vi "Initialize.vi"(8 "error in (no error)":errorcluster, 11 "State in":T1={"State"=enum."Idle", "Start Time"=timestamp(0 s since 1904-01-01), "Configuration"={"Cycle Period"=0.0, "PID 2 Parameters"={"Input Device"=enum."4-20mA", "Output Device"=enum."Default", "Setpoint"=0.0, "PID gains"={"proportional gain (Kc)"=0.0, "integral time (Ti, min)"=0.0, "derivative time (Td, min)"=100.0}, "output range"={"output low"=0.0, "output high"=1.0}}, "Manual Entry"=0.0, "Auto?"=TRUE, "4-20mA Input Settings"={"Input Channel "=0}, "4-20mA Out Settings"={"Output DAQ Task"=""}, "Input Channel Tag Name "=""}, "Current Time"=timestamp(0 s since 1904-01-01), "PID 1 Parameters"={"Setpoint"=0.0, "PID gains"={"proportional gain (Kc)"=1.0, "integral time (Ti, min)"=0.01, "derivative time (Td, min)"=0.0}}, "First Iteration"=FALSE, "Data"={"4-20mA Input"=0.0, "PID 2 Process Variable"=0.0, "PID 2 Output"=0.0, "4-20mA Output"=0.0}, "Process Name"="", "Pump On?"=enum."Off", "Input Error"=FALSE, "Output Error"=FALSE, "Log Started"=FALSE, "Current Setpoint"=0.0} {"Configuration"."PID 2 Parameters"."output range"."output low" format="%.2f"; "Configuration"."PID 2 Parameters"."output range"."output high" min=0.0 max=100.0 format="%.2f"; "Configuration"."PID 2 Parameters"."PID gains"."derivative time (Td, min)" format="%.3f"; "Configuration"."PID 2 Parameters"."PID gains"."integral time (Ti, min)" format="%.3f"; "Configuration"."PID 2 Parameters"."PID gains"."proportional gain (Kc)" format="%.3f"; "PID 1 Parameters"."PID gains"."derivative time (Td, min)" format="%.3f"; "PID 1 Parameters"."PID gains"."integral time (Ti, min)" format="%.3f"; "PID 1 Parameters"."PID gains"."proportional gain (Kc)" format="%.3f"}) -> (0 "error out":errorcluster, 1 "Pump Initialized":bool, 3 "State out":T1={"State"=enum."Idle", "Start Time"=timestamp(0 s since 1904-01-01), "Configuration"={"Cycle Period"=0.0, "PID 2 Parameters"={"Input Device"=enum."4-20mA", "Output Device"=enum."Default", "Setpoint"=0.0, "PID gains"={"proportional gain (Kc)"=0.0, "integral time (Ti, min)"=0.0, "derivative time (Td, min)"=100.0}, "output range"={"output low"=0.0, "output high"=1.0}}, "Manual Entry"=0.0, "Auto?"=TRUE, "4-20mA Input Settings"={"Input Channel "=0}, "4-20mA Out Settings"={"Output DAQ Task"=""}, "Input Channel Tag Name "=""}, "Current Time"=timestamp(0 s since 1904-01-01), "PID 1 Parameters"={"Setpoint"=0.0, "PID gains"={"proportional gain (Kc)"=1.0, "integral time (Ti, min)"=0.01, "derivative time (Td, min)"=0.0}}, "First Iteration"=FALSE, "Data"={"4-20mA Input"=0.0, "PID 2 Process Variable"=0.0, "PID 2 Output"=0.0, "4-20mA Output"=0.0}, "Process Name"="", "Pump On?"=enum."Off", "Input Error"=FALSE, "Output Error"=FALSE, "Log Started"=FALSE, "Current Setpoint"=0.0} {"Configuration"."PID 2 Parameters"."output range"."output low" format="%.2f"; "Configuration"."PID 2 Parameters"."output range"."output high" min=0.0 max=100.0 format="%.2f"; "Configuration"."PID 2 Parameters"."PID gains"."derivative time (Td, min)" format="%.3f"; "Configuration"."PID 2 Parameters"."PID gains"."integral time (Ti, min)" format="%.3f"; "Configuration"."PID 2 Parameters"."PID gains"."proportional gain (Kc)" format="%.3f"; "PID 1 Parameters"."PID gains"."derivative time (Td, min)" format="%.3f"; "PID 1 Parameters"."PID gains"."integral time (Ti, min)" format="%.3f"; "PID 1 Parameters"."PID gains"."proportional gain (Kc)" format="%.3f"})   [LabVIEW 2018, in "4-20mA Module.lvlib" / "4-20mA Module Engine.lvlib"]
uses:
  4-20mA Module Engine.lvlib
  State Cluster.ctl
  State Enum.ctl
  Pressure Transmitter/Pressure Transmitter Device Settings.ctl
  Pressure Reg Module/Pressure Regulator Device Settings.ctl
  Measure Instrument/PID 1 Parameters Cluster.ctl
  Tag VIs/Tag FGV Operation Enum.ctl
  Shared Variables/Dynamic Shared Variables.lvlib
  Pressure Transmitter/Pressure Transmitter Library.lvlib
  Pressure Reg Module/Pressure Regulator Library.lvlib
panel:
  # "Instrument Settings"
  # "Instrument Settings"
  # "Instrument Settings"
  # "Instrument Settings"
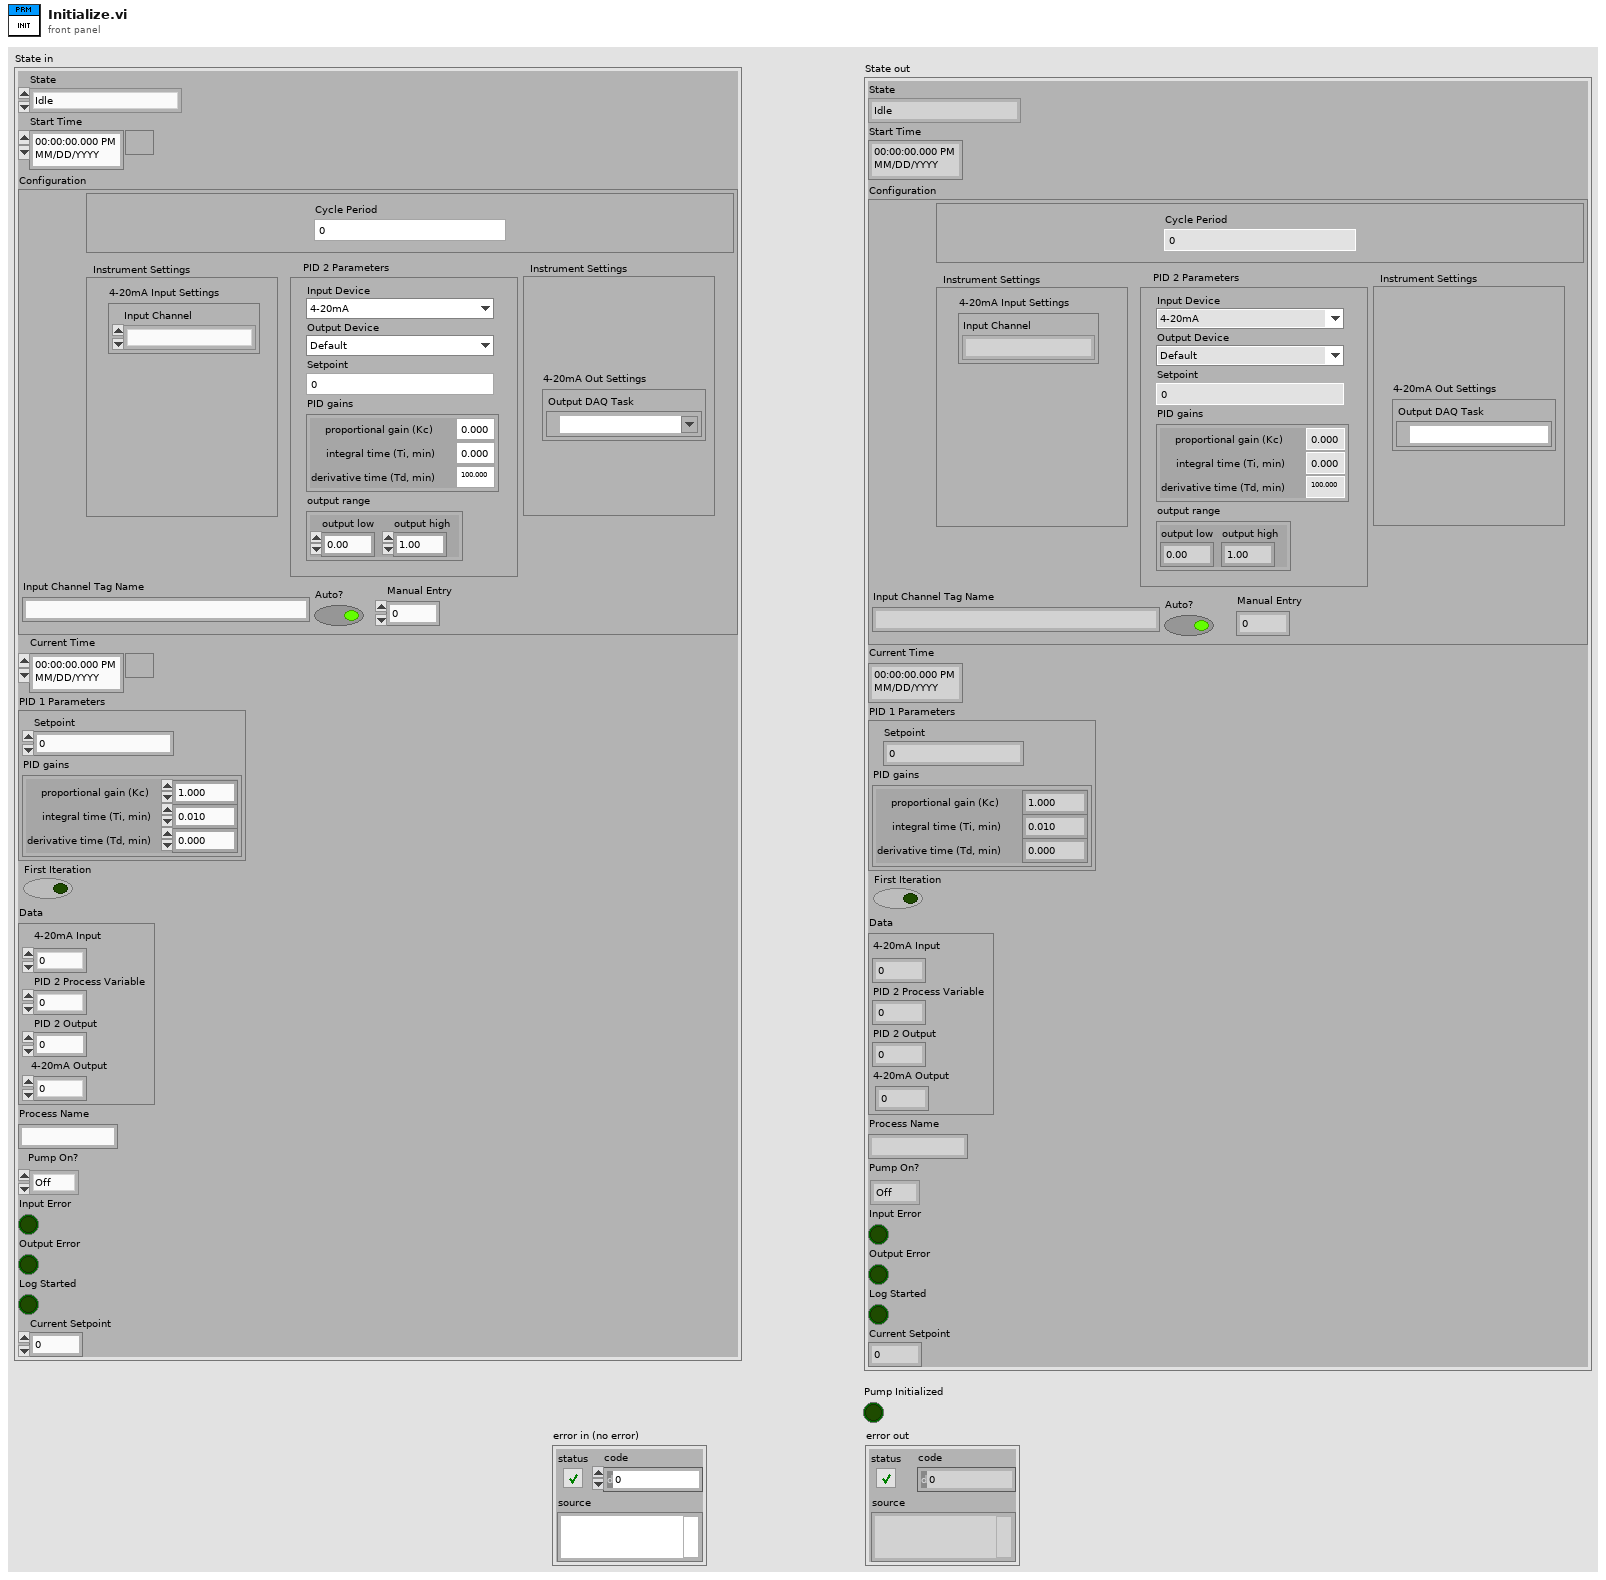
[diagram p1: front panel]
types:
  T1 = typedef "4-20mA Module.lvlib/4-20mA Module Engine.lvlib/State Cluster.ctl" = cluster{"State":T2, "Start Time":timestamp, "Configuration":cluster{"Cycle Period":dbl, "PID 2 Parameters":cluster{"Input Device":enum16{"Default", "4-20mA"}, "Output Device":enum16{"Default", "Equilibar Pressure Reg", "Flow Regulator"}, "Setpoint":dbl, "PID gains":cluster{"proportional gain (Kc)":dbl, "integral time (Ti, min)":dbl, "derivative time (Td, min)":dbl}, "output range":cluster{"output low":dbl, "output high":dbl}}, "Manual Entry":dbl, "Auto?":bool, "4-20mA Input Settings":T3, "4-20mA Out Settings":T4, "Input Channel Tag Name ":string}, "Current Time":timestamp, "PID 1 Parameters":T5, "First Iteration":bool, "Data":cluster{"4-20mA Input":dbl, "PID 2 Process Variable":dbl, "PID 2 Output":dbl, "4-20mA Output":dbl}, "Process Name":string, "Pump On?":enum16{"Off", "On", "Not Initialized"}, "Input Error":bool, "Output Error":bool, "Log Started":bool, "Current Setpoint":dbl}
  T2 = typedef "4-20mA Module.lvlib/4-20mA Module Engine.lvlib/State Enum.ctl" = enum16{"Measuring", "Idle", "Paused"}
  T3 = typedef "Pressure Transmitter Library.lvlib/Pressure Transmitter Device Settings.ctl" = cluster{"Input Channel ":u16}
  T4 = typedef "Pressure Regulator Library.lvlib/Pressure Regulator Device Settings.ctl" = cluster{"Output DAQ Task":refnum<k21>}
  T5 = typedef "PID 1 Parameters Cluster.ctl" = cluster{"Setpoint":dbl, "PID gains":cluster{"proportional gain (Kc)":dbl, "integral time (Ti, min)":dbl, "derivative time (Td, min)":dbl}}
  T6 = typedef "Tag FGV Operation Enum.ctl" = enum16{"Init", "Set Notification Queue", "Create Tag", "Commit", "Write Tag (Numeric)", "Write Tag (Boolean)", "Read All Tags", "Read One Tag", "Delete Tag Category", "Set Alarm Parameters (Numeric)", "Set Alarm Parameters (Boolean)", "Enable All Alarms", "Disable All Alarms", "Delete All Tags", "Read Alarms", "Ack Alarm", "Read Alarm Parameters (Numeric)", "Read Alarm Parameters (Boolean)"}
  T7 = enum16{"Default", "Equilibar Pressure Reg", "Flow Regulator"}
  T8 = typedef "4-20mA Module.lvlib/4-20mA Module Tag Names Cluster.ctl" = cluster{"4-20mA Input":string, "PID 2 Out Tag":string, "4-20mA Output":string, "Input Device Tag":string, "Output Device Tag":string}
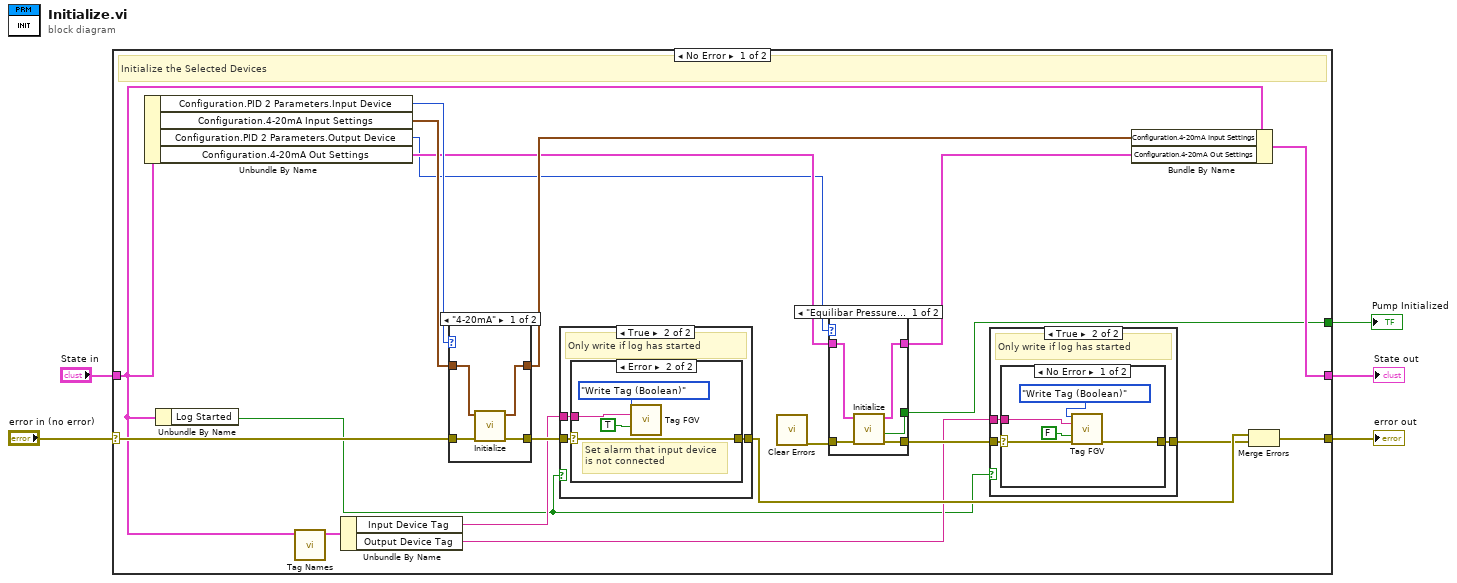
[diagram p0: block diagram]
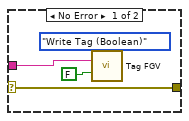
[diagram p3: hidden frame]
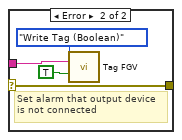
[diagram p5: hidden frame]
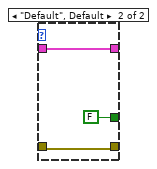
[diagram p6: hidden frame]
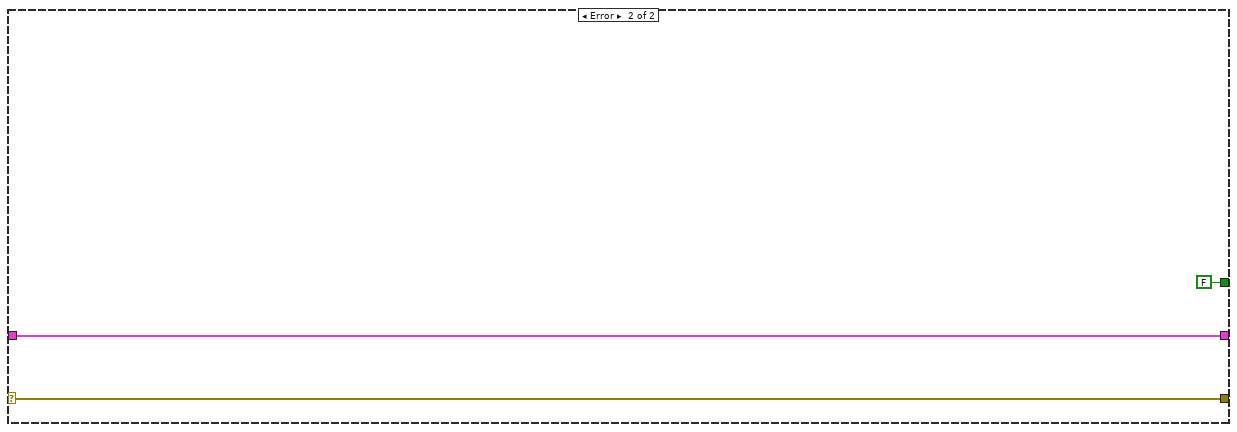
[diagram p8: hidden frame]
diagram:
  n1 = case shown="No Error" "error in (no error)" {
    selector: "error in (no error)" -> [w23 w67]
    tunnel: [w14 w67] -> w4
    tunnel: "State in" -> [w7 w66]
    tunnel: [w22 w66] -> w2
    tunnel: [w9 FALSE ("Initialized")] -> w1
    frame No Error {
      # "Initialize the Selected Devices"
      n2 = Unbundle By Name(w7) -> ("Configuration.PID 2 Parameters.Input Device"=w25:enum16{"Default", "4-20mA"}, "Configuration.4-20mA Input Settings"=w24:T3, "Configuration.PID 2 Parameters.Output Device"=w10:T7, "Configuration.4-20mA Out Settings"=w20:T4)
      n3 = Unbundle By Name(w7) -> ("Log Started"=w8:bool)
      n4 = call "Tag Names.vi"("State in"=w7) -> ("4-20mA Module Tag Names"=w18:T8)  [unwired: 8 in, 2 out]
      n5 = Unbundle By Name(w18) -> ("Input Device Tag"=w17:string, "Output Device Tag"=w11:string)
      n6 = case shown="\"4-20mA\"" w25 {
        tunnel: w24 -> [w60 w64]
        tunnel: w23 -> [w62 w63]
        tunnel: [w61 w63] -> w19
        tunnel: [w59 w64] -> w21
        frame "4-20mA" {
          n7 = call "Initialize.vi"("error in"=w62, "4-20mA Settings In"=w60) -> ("error out"=w61:errorcluster, "4-20mA Settings Out"=w59:T3)  [unwired: 7 in, 1 out]
        }
        frame "Default", Default {
        }
      }
      n8 = case shown="True" w8 {
        tunnel: w19 -> [w26 w29]
        tunnel: w17 -> [_ w28]
        tunnel: [w26 w27] -> w16
        frame False {
        }
        frame True {
          # "Only write if log has started"
          n9 = case shown="Error" w29 {
            selector: w29 -> [w30 w35]
            tunnel: [w30 w35] -> w27
            tunnel: w28 -> [w31 w34]
            frame No Error {
              n10 = call "Tag FGV.vi"("Operation"=Tag_FGV_Operation_Enum."Write Tag (Boolean)", "Tag Name"=w31, "Data"=FALSE) -> ()  [unwired: 5 in, 8 out]
            }
            frame Error {
              # "Set alarm that input device\nis not connected"
              n11 = call "Tag FGV.vi"("Operation"=Tag_FGV_Operation_Enum."Write Tag (Boolean)", "Tag Name"=w34, "Data"=TRUE) -> ()  [unwired: 5 in, 8 out]
            }
          }
        }
      }
      n12 = call <vilib>:"Clear Errors.vi"() -> ("error out"=w15:errorcluster)  [unwired: 6 in, 1 out]
      n13 = case shown="\"Equilibar Pressure Reg\"" w10 {
        tunnel: w20 -> [w52 w58]
        tunnel: [w51 w58] -> w6
        tunnel: w15 -> [w55 w57]
        tunnel: [w54 w57] -> w13
        tunnel: [w53 FALSE ("Initialized")] -> w9
        frame "Equilibar Pressure Reg" {
          n14 = call "Initialize.vi"("error in"=w55, "4-20mA Out Settings In"=w52) -> ("error out"=w54:errorcluster, "Initialized"=w53:bool, "4-20mA Out Settings Out"=w51:T4)  [unwired: 7 in]
        }
        frame "Default", Default {
        }
      }
      n15 = case shown="True" w8 {
        tunnel: w13 -> [w38 w41]
        tunnel: [w38 w40] -> w12
        tunnel: w11 -> [_ w39]
        frame False {
        }
        frame True {
          # "Only write if log has started"
          n16 = case shown="No Error" w41 {
            selector: w41 -> [w43 w48]
            tunnel: [w42 w48] -> w40
            tunnel: w39 -> [w44 w47]
            frame No Error {
              n17 = call "Tag FGV.vi"("Operation"=Tag_FGV_Operation_Enum."Write Tag (Boolean)", "Tag Name"=w44, "Data"=FALSE, "error in (no error)"=w43) -> ("error out"=w42:errorcluster)  [unwired: 4 in, 7 out]
            }
            frame Error {
              # "Set alarm that output device\nis not connected"
              n18 = call "Tag FGV.vi"("Operation"=Tag_FGV_Operation_Enum."Write Tag (Boolean)", "Tag Name"=w47, "Data"=TRUE) -> ()  [unwired: 5 in, 8 out]
            }
          }
        }
      }
      n19 = Bundle By Name(cluster=w7, "Configuration.4-20mA Input Settings"=w21, "Configuration.4-20mA Out Settings"=w6) -> (w22:T1)
      n20 = Merge Errors(w16, w12) -> (w14:errorcluster)
    }
    frame Error {
    }
  }
  "error out" <- w4
  "State out" <- w2
  "Pump Initialized" <- w1
